vi "Close DB.vi"(8 "error in (no error)":errorcluster, 11 "NI_DB_API in":refnum<class "NI_DB_API.lvclass">) -> (0 "error out":errorcluster, 3 "NI_DB_API out":refnum<class "NI_DB_API.lvclass">)   [LabVIEW 2021, in "NI_DB_API.lvclass"]
uses:
  <userlib>/John_Lib/DataBase/NI_DB_API/NI_DB_API.lvclass
  <userlib>/John_Lib/DataBase/NI_DB_API/NI_DB_API.lvclass/NI_DB_API.ctl
  <vilib>/addons/database/NI_Database_API.lvlib
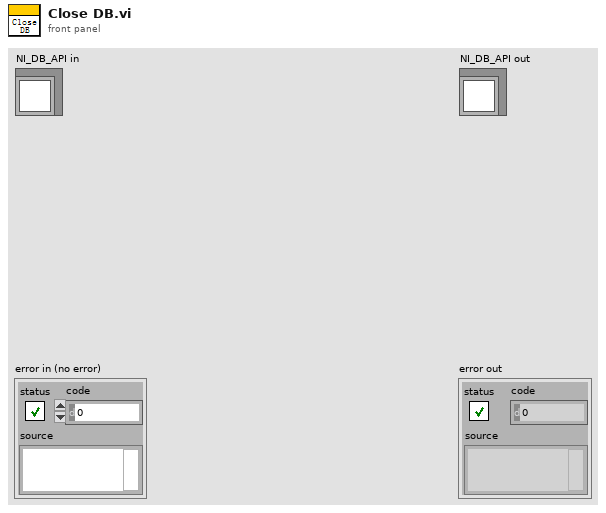
[diagram p1: front panel]
types:
  T1 = typedef "NI_Database_API.lvlib/Conn ObjectReference.ctl" = refnum<k1>
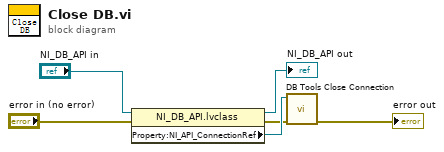
[diagram p0: block diagram]
diagram:
  n1 = property class="NI_DB_API.lvclass"(reference="NI_DB_API in", error in="error in (no error)") -> (reference out=→"NI_DB_API out":refnum<class "NI_DB_API.lvclass">, error out=w4:errorcluster, "Property:NI_API_ConnectionRef"=w5:T1)
  n2 = call <vilib>:"DB Tools Close Connection.vi"("error in (no error)"=w4, "connection reference"=w5) -> ("error out"=→"error out":errorcluster)  [unwired: 5 in]
